vi "AddLimit.vi"(7 "ComparisonType":T1, 8 "error in":errorcluster, 9 "HigherBound":timestamp, 10 "LowerBound":timestamp, 11 "DateTimeMeasure in":refnum<class "DateTimeMeasure.lvclass">) -> (0 "error out":errorcluster, 2 "DateTimeMeasureLimit":refnum<class "DateTimeMeasureLimit.lvclass">, 3 "DateTimeMeasure out":refnum<class "DateTimeMeasure.lvclass">)   [LabVIEW 2021, in "ProligentXMLGenerator.lvlib" / "DateTimeMeasure.lvclass"]
doc: "Add a MeasureLimit element.\n\nThe limit expression associated with the measure."
uses:
  DateTimeMeasure.lvclass
  DateTimeMeasure.lvclass/DateTimeMeasure.ctl
  MeasureLimit/MeasureLimit.lvclass
  DateTimeMeasureLimit/DateTimeMeasureLimit.lvclass
  RangeMeasureLimit/ComparisonType.ctl
  RangeMeasureLimit/RangeMeasureLimit.lvclass
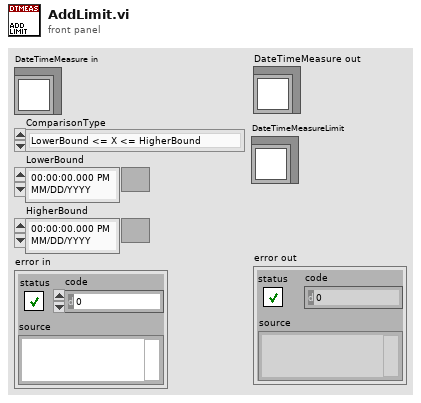
[diagram p1: front panel]
types:
  T1 = typedef "ProligentXMLGenerator.lvlib/RangeMeasureLimit.lvclass/ComparisonType.ctl" = enum16{"LowerBound <= X <= HigherBound", "LowerBound < X <= HigherBound", "LowerBound <= X < HigherBound", "LowerBound < X < HigherBound", "LowerBound <= X", "LowerBound < X", "X <= HigherBound", "X < HigherBound", "X == HigherBound", "X != HigherBound", "X <= LowerBound OR HigherBound <= X", "X < LowerBound OR HigherBound <= X", "X <= LowerBound OR HigherBound < X", "X < LowerBound OR HigherBound < X"}
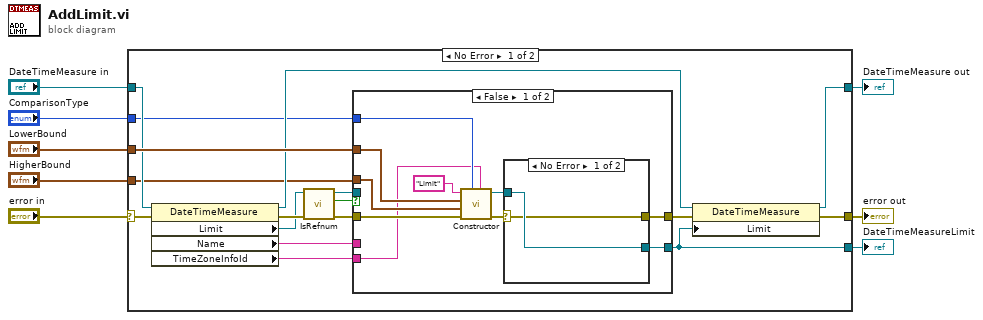
[diagram p0: block diagram]
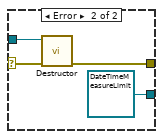
[diagram p2: hidden frame]
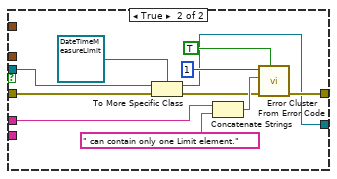
[diagram p3: hidden frame]
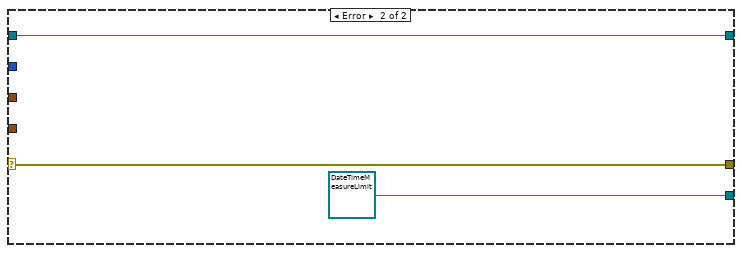
[diagram p4: hidden frame]
diagram:
  n1 = case shown="No Error" "error in" {
    selector: "error in" -> [w24 w54]
    tunnel: [w16 refnum<class "DateTimeMeasureLimit.lvclass"> refnum ("ProligentResultProcessor:DateTimeMeasureLimit")] -> w4
    tunnel: [w18 w54] -> w7
    tunnel: "DateTimeMeasure in" -> [w15 w55]
    tunnel: [w17 w55] -> w5
    tunnel: "LowerBound" -> [w19 _]
    tunnel: "ComparisonType" -> [w11 _]
    tunnel: "HigherBound" -> [w10 _]
    frame No Error {
      n2 = property class="DateTimeMeasure"(reference=w15, error in=w24) -> (reference out=w14:refnum<class "DateTimeMeasure.lvclass">, error out=w23:errorcluster, "Limit"=w13:refnum<class "MeasureLimit.lvclass">, "Name"=w22:string, "TimeZoneInfoId"=w9:string)
      n3 = call "IsRefnum.vi"("error in"=w23, "MeasureLimit in"=w13) -> ("error out"=w21:errorcluster, "IsRefnum"=w20:bool, "MeasureLimit out"=w12:refnum<class "MeasureLimit.lvclass">)  [unwired: 7 in]
      n4 = case shown="False" w20 {
        tunnel: w21 -> [w32 w45]
        tunnel: [w35 w48] -> w25
        tunnel: [w34 w43] -> w16
        tunnel: w22 -> [_ w47]
        tunnel: w19 -> [w29 _]
        tunnel: w12 -> [_ w46]
        tunnel: w11 -> [w28 _]
        tunnel: w10 -> [w27 _]
        tunnel: w9 -> [w26 _]
        frame False {
          n5 = call "Constructor.vi"("TimeZoneInfoId"=w26, "ComparisonType"=w28, "error in"=w32, "HigherBound"=w27, "LowerBound"=w29, "Name"="Limit") -> ("error out"=w31:errorcluster, "DateTimeMeasureLimit"=w30:refnum<class "DateTimeMeasureLimit.lvclass">)  [unwired: 4 in]
          n6 = case shown="No Error" w31 {
            selector: w31 -> [w36 w41]
            tunnel: w30 -> [w37 w39]
            tunnel: [w36 w40] -> w35
            tunnel: [w37 refnum<class "DateTimeMeasureLimit.lvclass"> refnum ("BooleanMeasureLimit")] -> w34
            frame No Error {
            }
            frame Error {
              n7 = call "Destructor.vi"("error in"=w41, "DateTimeMeasureLimit"=w39) -> ("error out"=w40:errorcluster)  [unwired: 9 in]
            }
          }
        }
        frame True {
          n8 = To More Specific Class(target class=refnum<class "DateTimeMeasureLimit.lvclass"> refnum ("ProligentResultProcessor:DateTimeMeasureLimit"), reference=w46, error in=w45) -> (specific class reference=w43:refnum<class "DateTimeMeasureLimit.lvclass">, error out=w44:errorcluster)
          n9 = Concatenate Strings(w47, " can contain only one Limit element." ("string")) -> (w52:string)
          n10 = call <vilib>:"Error Cluster From Error Code.vi"("show call chain? (False)"=TRUE, "error in (no error)"=w44, "error message (\"\")"=w52, "error code (0)"=1) -> ("error out"=w48:errorcluster)  [unwired: 5 in]
        }
      }
      n11 = property class="DateTimeMeasure"(reference=w14, error in=w25, "Limit"=w16) -> (reference out=w17:refnum<class "DateTimeMeasure.lvclass">, error out=w18:errorcluster)
    }
    frame Error {
    }
  }
  "error out" <- w7
  "DateTimeMeasure out" <- w5
  "DateTimeMeasureLimit" <- w4
